vi "Simon_JKI.vi"() -> ()   [LabVIEW 2020]
uses:
  Simon Properties.ctl
  Tab Control.ctl
  <vilib>/Utility/file.llb/Read Delimited Spreadsheet (string).vi
  <vilib>/Utility/file.llb/Write Delimited Spreadsheet (string).vi
  Login Button.ctl
  Signin Button.ctl
panel:
  out "login status":string
  in  "OK":bool
  in  "Tab Control":T1
  in  "Quick Start":bool
  in  "Signin Button":T2
  in  "Login Button":T3 caption="OK Button"
  in  "Log in confirm":bool
  in  "请输入账号":string caption="Please enter your account:"
  in  "请输入密码":string caption="Please enter your password:"
  in  "请输入账号注册":string caption="Please enter your account:"
  in  "请输入密码注册":string caption="Please enter your password:"
  in  "Sign in Confirm":bool
  in  "Please enter your answer:":T4
  out "Sequence for Player to Memorize":u32(colorbox)
  out "The numbe of colors \nyou have memorized!":i32
  in  "Level Confirm":bool
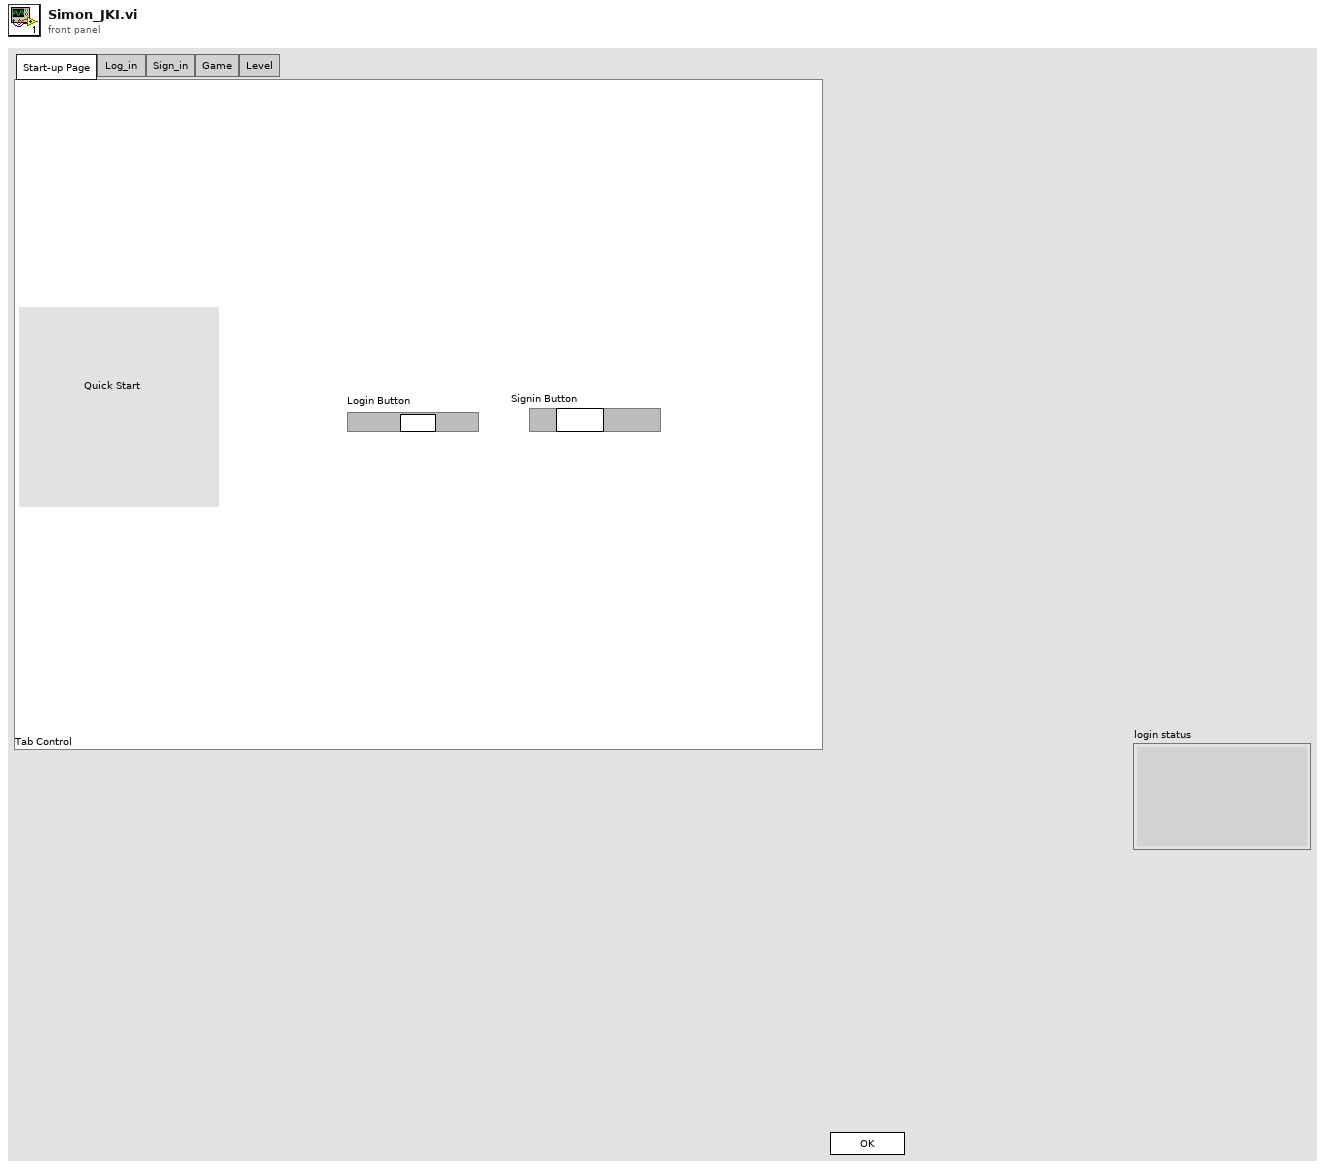
[diagram p1: front panel]
types:
  T1 = typedef "Tab Control.ctl" = enum32{"Start-up Page", "Log_in ", "Sign_in", "Game", "Level"}
  T2 = typedef "Signin Button.ctl" = bool
  T3 = typedef "Login Button.ctl" = bool
  T4 = cluster{"0":bool, "7":bool, "8":bool, "9":bool, "4":bool, "5":bool, "6":bool, "1":bool, "2":bool, "3":bool}
  T5 = enum32{"Invalid", "Standard", "Closed", "Hidden", "Minimized", "Maximized"}
  T6 = enum32{"invalid app kind", "Development System", "Run Time System", "Student Edition", "Embedded LabVIEW", "Evaluation", "Custom"}
  T7 = typedef "Simon Properties.ctl" = cluster{"Sequence ":i32[], "\n Colors":u32[], "Wait Time (ms)":u32, "Last Key":i16, "Number of Key Pressed":i32, "Record\n":i32, "Log_in":bool}
  T8 = cluster{"Core":cluster{"Current VI Reference":refnum<vi>, "Close Panel on Exit?":bool}, "Simon Properties":T7}
  T9 = cluster{"Current VI Reference":refnum<vi>, "Close Panel on Exit?":bool}
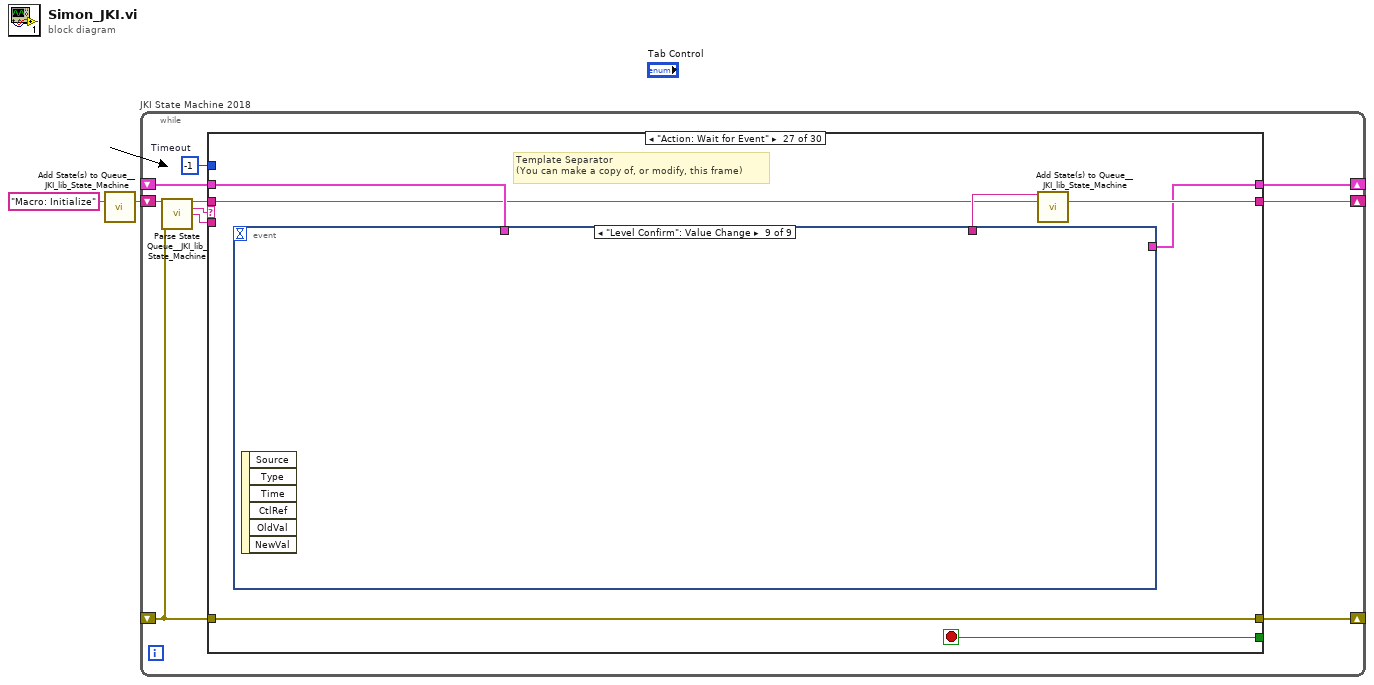
[diagram p0: block diagram]
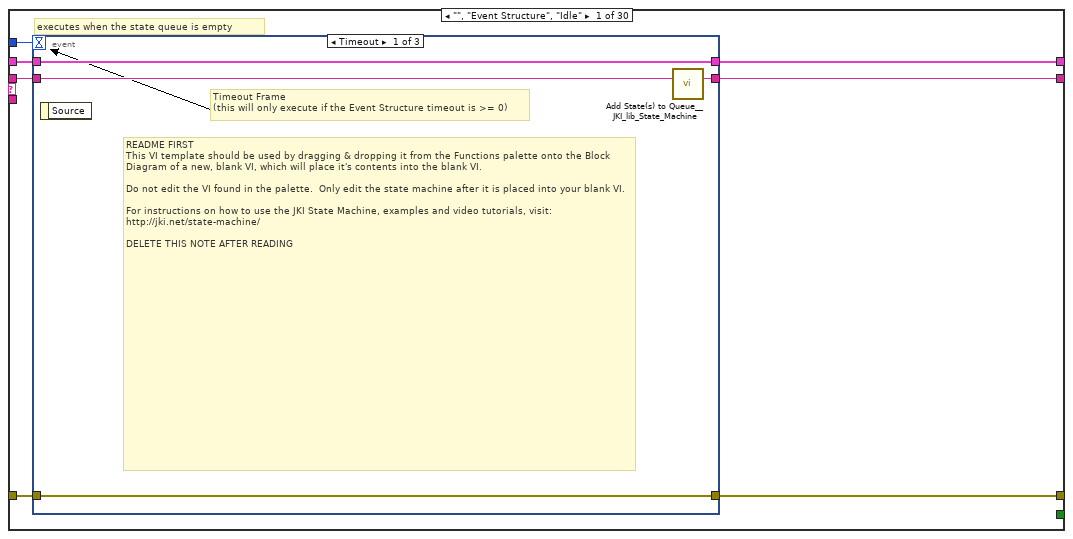
[diagram p2: hidden frame]
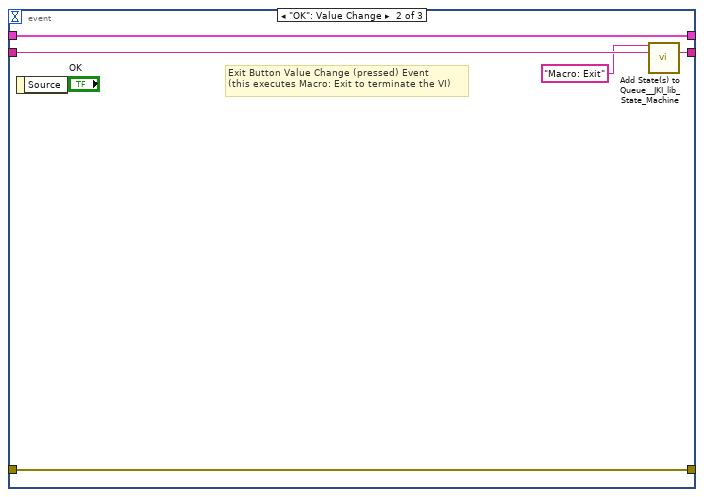
[diagram p3: hidden frame]
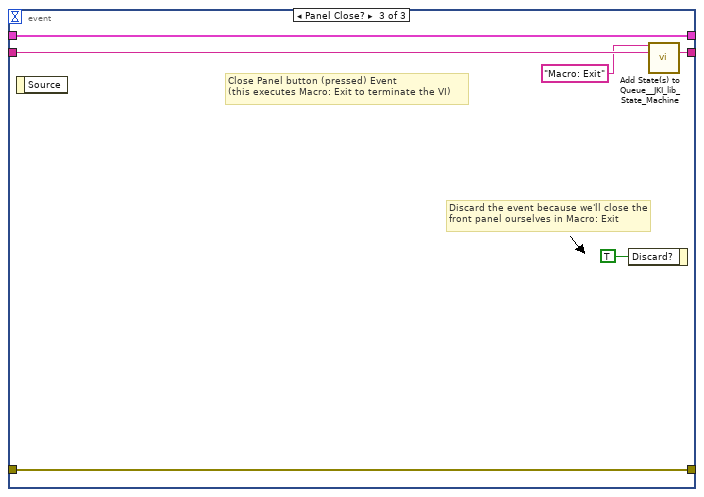
[diagram p4: hidden frame]
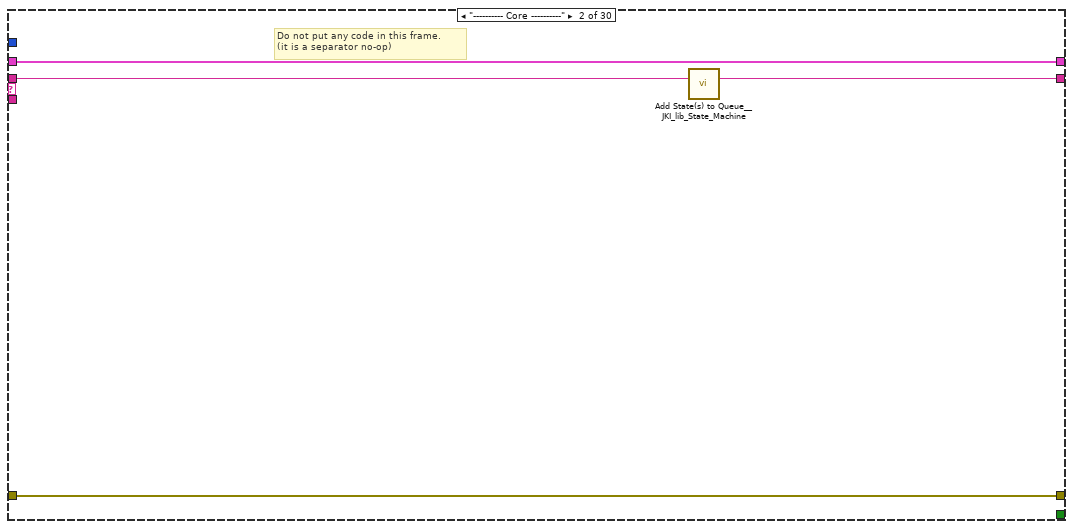
[diagram p5: hidden frame]
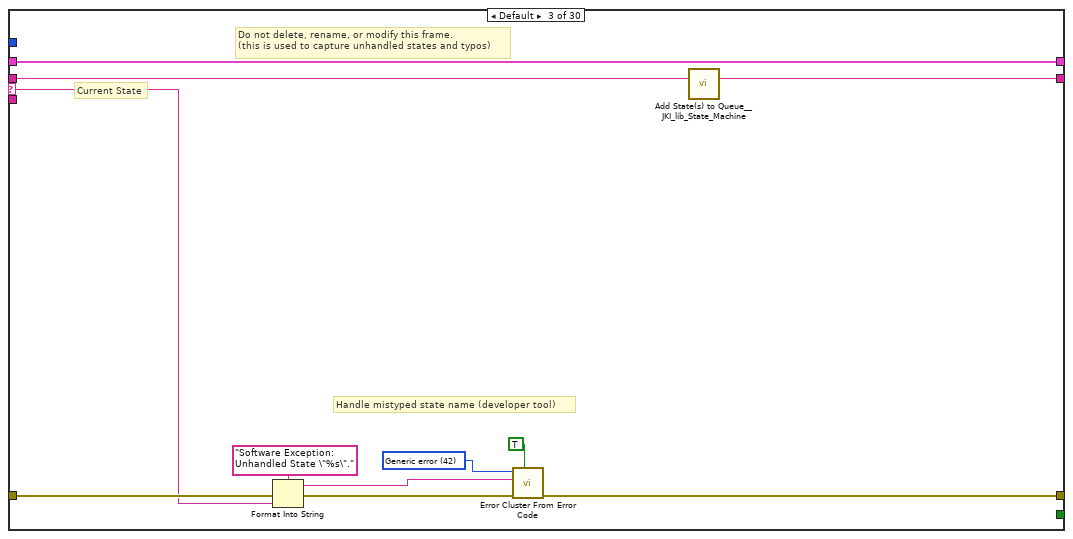
[diagram p6: hidden frame]
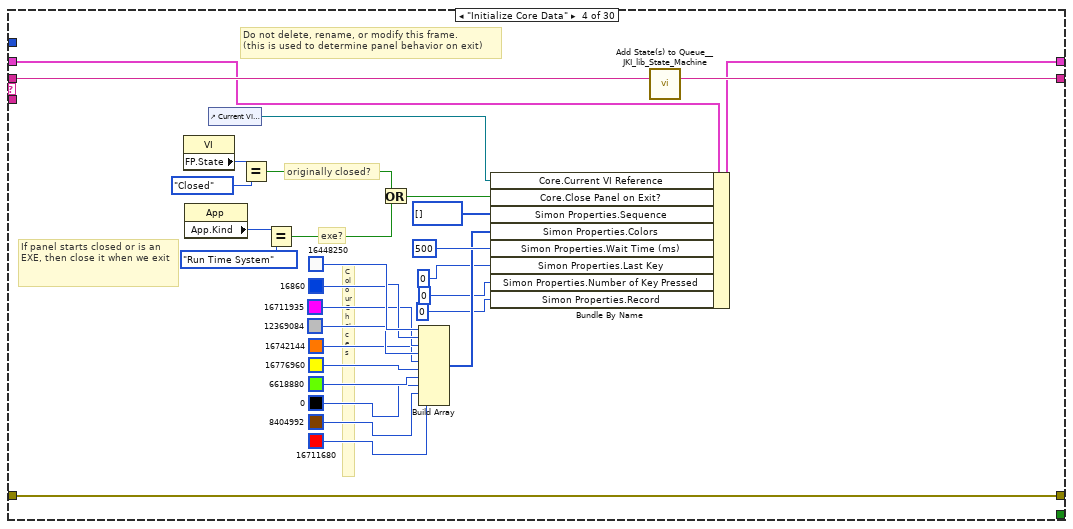
[diagram p7: hidden frame]
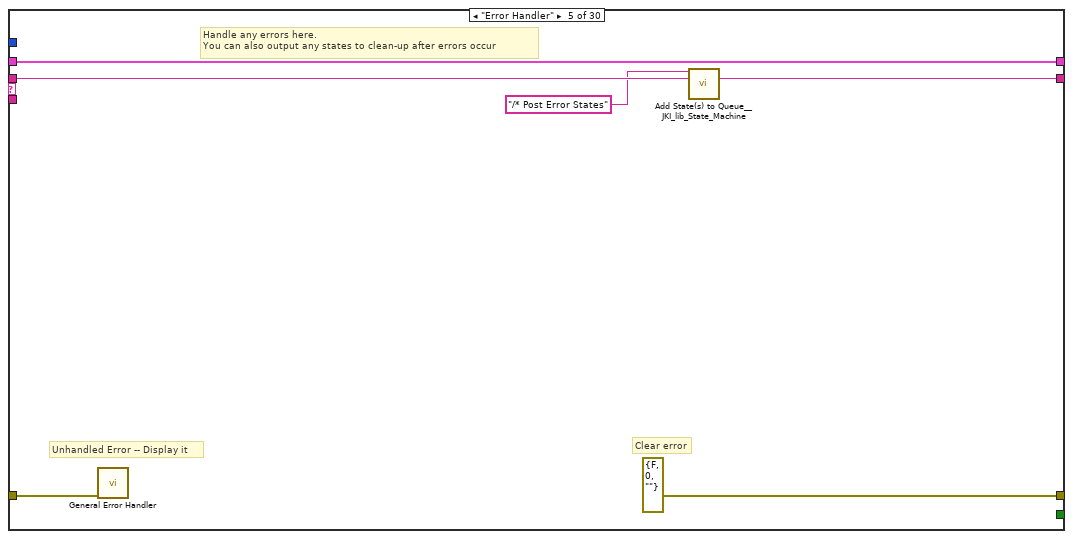
[diagram p8: hidden frame]
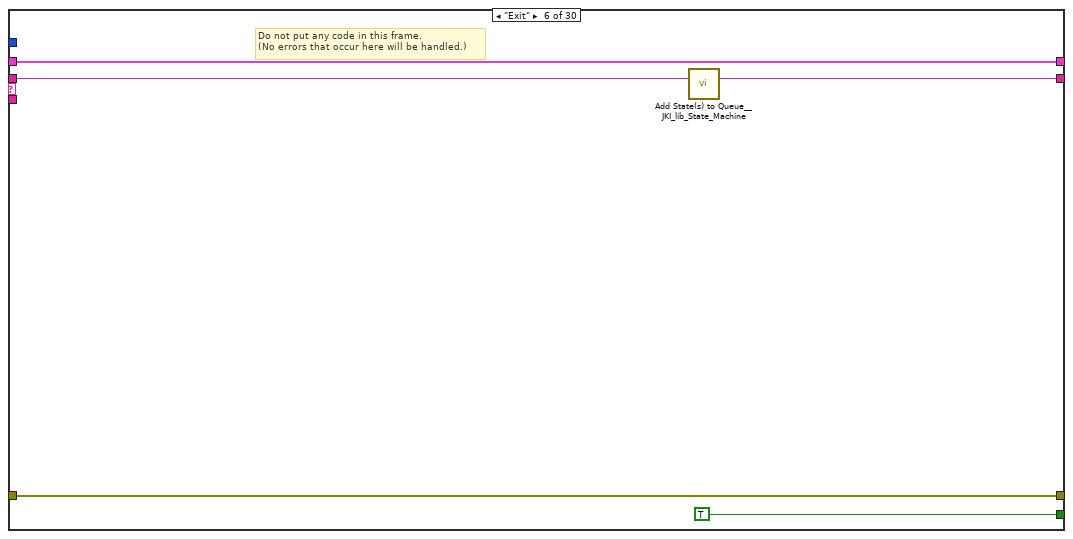
[diagram p9: hidden frame]
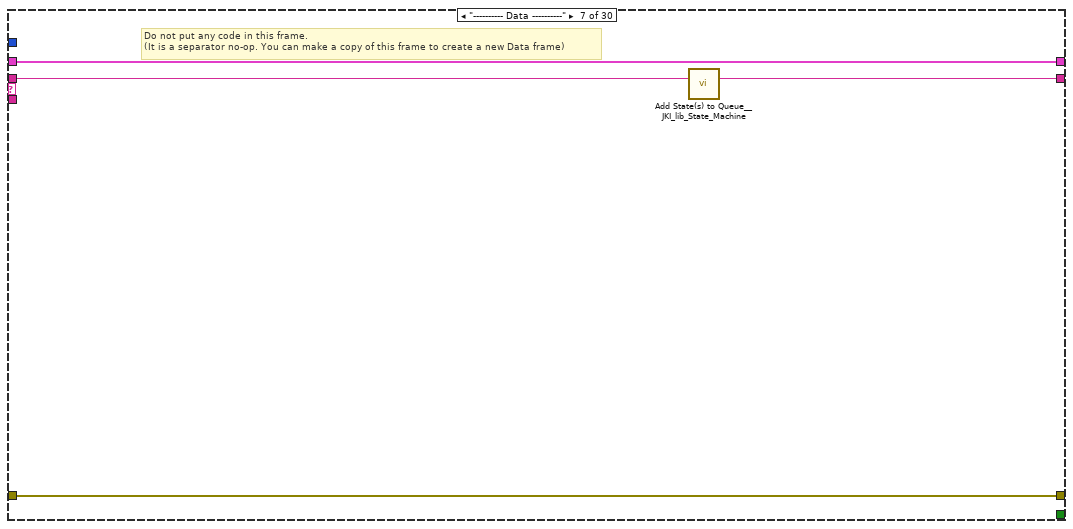
[diagram p10: hidden frame]
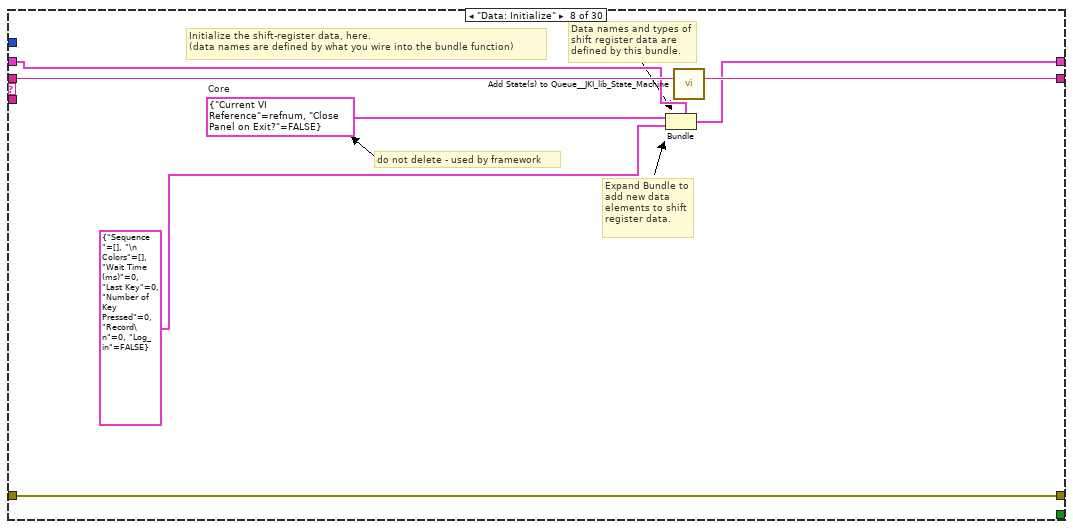
[diagram p11: hidden frame]
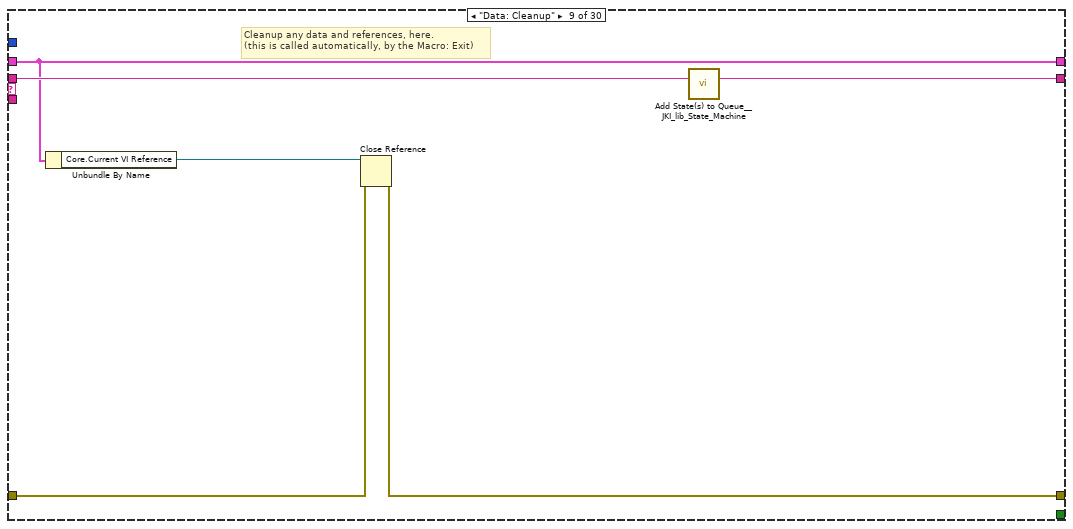
[diagram p12: hidden frame]
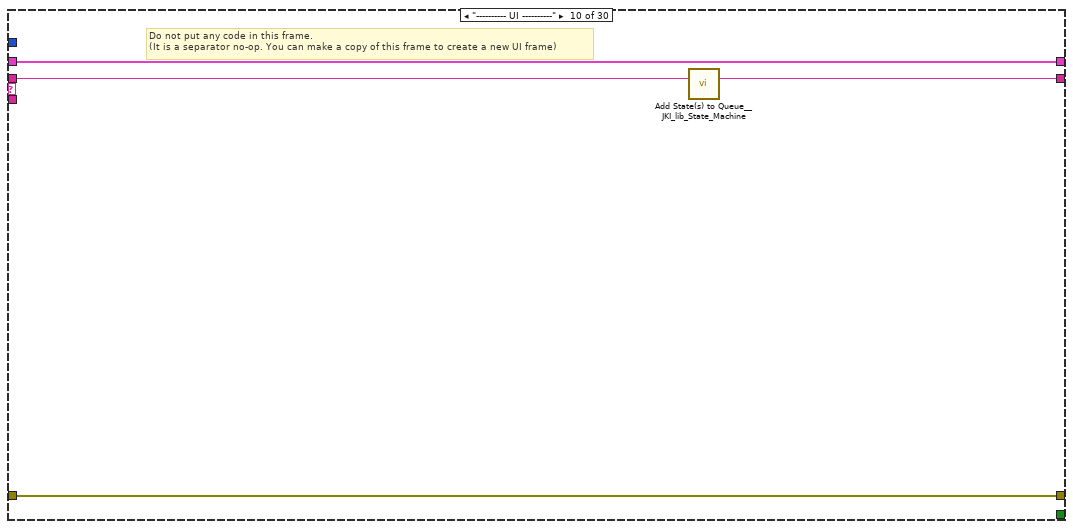
[diagram p13: hidden frame]
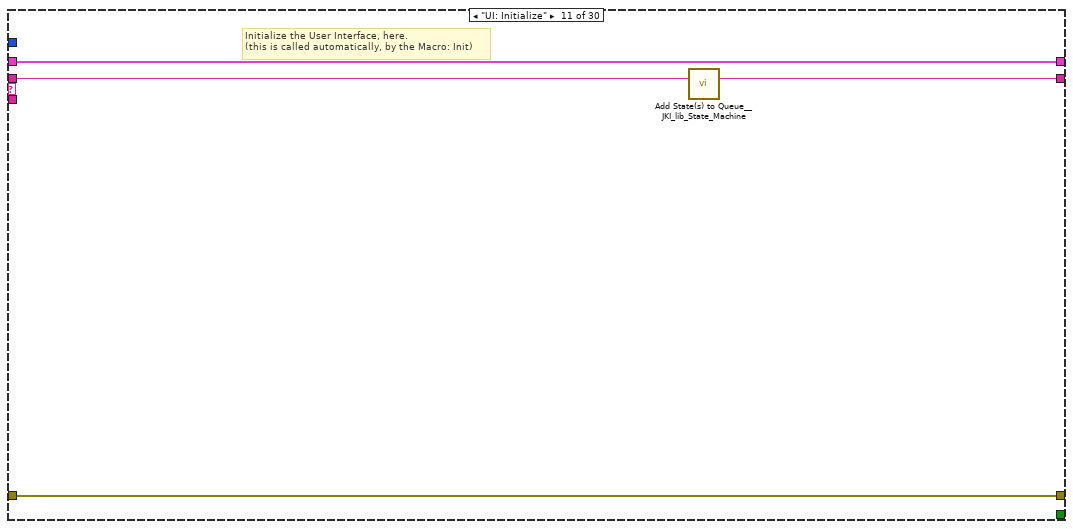
[diagram p14: hidden frame]
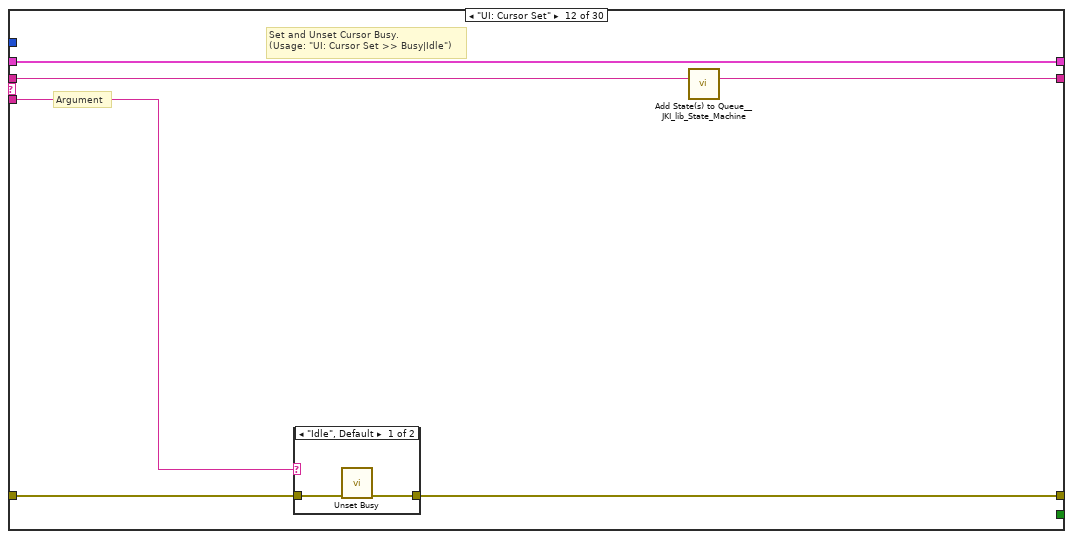
[diagram p15: hidden frame]
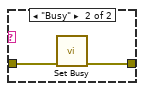
[diagram p16: hidden frame]
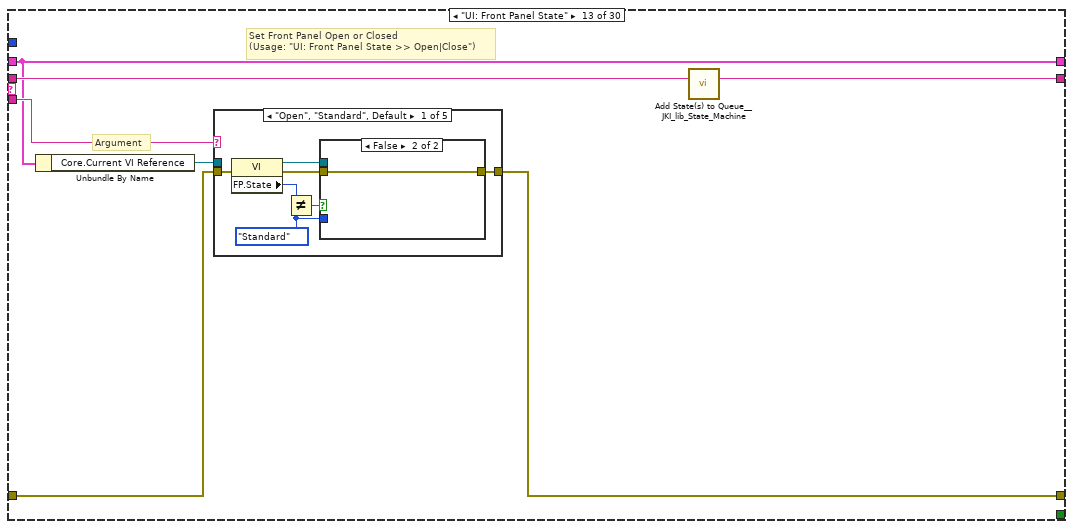
[diagram p17: hidden frame]
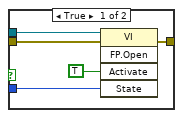
[diagram p18: hidden frame]
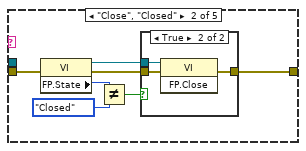
[diagram p19: hidden frame]
diagram:
  n1 = call <vilib>:"Add State(s) to Queue__JKI_lib_State_Machine.vi"("State(s) in (\"\")"="Macro: Initialize") -> ("States Out"=w2:string)  [unwired: 14 in]
  n2 = while "JKI State Machine 2018" {
    shift-right: [w6] -> _
    shift-left: _ -> [w5]
    shift-right: [w9] -> _
    shift-left: _ -> [w3]
    shift-right: [w8] -> _
    shift-left: w2 -> [w10]
    stop <- w7 stop-if-true
    w4 = -1  # Timeout
    n3 = call <vilib>:"Parse State Queue__JKI_lib_State_Machine.vi"("State Queue"=w10, "Error In (no error)"=w3) -> ("Remaining States"=w12:string, "Current State"=w13:string, "Arguments"=w11:string)  [unwired: 11 in]
    n4 = case shown="\"Action: Wait for Event\"" w13 {
      selector: w13 -> [_ _ w40 _ _ _ _ _ _ _ _ _ _ _ _ _ _ _ _ _ _ _ _ _ _ _ _ _ _ _]
      tunnel: w12 -> [w20 w39 w44 w79 w85 w90 w94 w101 w107 w111 w115 w121 w132 w196 w201 w206 w216 w220 w224 w229 w237 w243 w247 w253 w261 w284 w293 w369 w386 w394]
      tunnel: w11 -> [_ _ _ _ _ _ _ _ _ _ _ w116 w127 _ _ _ _ _ _ _ _ _ _ _ _ _ _ _ _ _]
      tunnel: w5 -> [w18 w36 w42 w58 w82 w88 w91 w96 w102 w108 w113 w119 w126 w193 w198 w203 w207 w217 w225 w231 w238 w244 w248 w254 w262 w282 w297 w371 w384 w396]
      tunnel: [w17 w37 w46 w77 errorcluster {"status"=FALSE, "code"=0, "source"=""} ("error out") w87 w92 w99 w104 w109 w112 w117 w129 w194 w199 w204 w214 w218 w222 w227 w234 w240 _ w250 w259 w281 w294 w367 w382 w393] -> w9
      tunnel: w3 -> [w16 w37 w45 w77 w81 w87 w92 w99 w105 w109 w112 w118 w130 w194 w199 w204 w214 w218 w222 w227 w234 w240 _ w250 w259 w281 w294 w367 w382 w393]
      tunnel: [w19 w38 w43 w78 w84 w89 w93 w100 w106 w110 w114 w120 w131 w195 w200 w205 w215 w219 w223 w228 w235 w241 w246 w252 w260 w283 w296 w368 w385 w395] -> w8
      tunnel: [_ _ _ _ _ TRUE _ _ _ _ _ _ _ _ _ _ _ _ _ _ _ _ _ _ _ _ _ _ _ _] -> w7
      tunnel: [w15 w36 w42 w57 w82 w88 w91 w95 w102 w108 w113 w119 w126 w193 w198 w203 w207 w217 w225 w231 w238 w244 w248 w254 w263 w282 w295 w370 w387 w396] -> w6
      tunnel: w4 -> [w14 _ _ _ _ _ _ _ _ _ _ _ _ _ _ _ _ _ _ _ _ _ _ _ _ _ _ _ _ _]
      frame "", "Event Structure", "Idle" {
        # "executes when the state queue is empty"
        n5 = event shown="[0] Timeout" {
          selector: _ -> [_ _ _]
          dyn-events: _ -> [_ _ _]
          timeout: w14 -> [_ _ _]
          tunnel: w20 -> [w24 w29 w35]
          tunnel: [w23 w28 w34] -> w19
          tunnel: w18 -> [w21 w26 w32]
          tunnel: [w22 w27 w33] -> w17
          tunnel: w16 -> [w22 w27 w33]
          tunnel: [w21 w26 w32] -> w15
          event Timeout {
            # "README FIRST\nThis VI template should be used by dragging & dropping it from the Functions palette onto the Block Diagram of a new, blank VI, which will place it's contents into the blank VI.\n\nDo not edit the VI found in the palette.  Only edit the state machine after it is placed into your blank VI.\n\nFor instructions on how to use the JKI State Machine, examples and video tutorials, visit:\nhttp://jki.net/state-machine/\n\nDELETE THIS NOTE AFTER READING"
            # "Timeout Frame\n(this will only execute if the Event Structure timeout is >= 0)"
            n6 = event-data() -> ()  [unwired: 1 in, 1 out]
            n7 = call <vilib>:"Add State(s) to Queue__JKI_lib_State_Machine.vi"("State(s) in (\"\")"=w24) -> ("States Out"=w23:string)  [unwired: 14 in]
          }
          event "OK": Value Change {
            # "Exit Button Value Change (pressed) Event\n(this executes Macro: Exit to terminate the VI)"
            n8 = event-data() -> ()  [unwired: 1 in, 1 out]
            n9 = call <vilib>:"Add State(s) to Queue__JKI_lib_State_Machine.vi"("State(s) in Front (\"\")"="Macro: Exit", "State(s) in (\"\")"=w29) -> ("States Out"=w28:string)  [unwired: 13 in]
          }
          event Panel Close? {
            # "Discard the event because we'll close the front panel ourselves in Macro: Exit"
            # "Close Panel button (pressed) Event\n(this executes Macro: Exit to terminate the VI)"
            n10 = event-data() -> ()  [unwired: 1 in, 1 out]
            n11 = event-data("Discard?"=TRUE) -> ()  [unwired: 1 in, 1 out]
            n12 = call <vilib>:"Add State(s) to Queue__JKI_lib_State_Machine.vi"("State(s) in Front (\"\")"="Macro: Exit", "State(s) in (\"\")"=w35) -> ("States Out"=w34:string)  [unwired: 13 in]
          }
        }
      }
      frame "---------- Core ----------" {
        # "Do not put any code in this frame.\n(it is a separator no-op)"
        n13 = call <vilib>:"Add State(s) to Queue__JKI_lib_State_Machine.vi"("State(s) in (\"\")"=w39) -> ("States Out"=w38:string)  [unwired: 14 in]
      }
      frame Default {
        w49 = 42 items=["No error", "Argument error", "Memory is full", "Out of zone", "End of file", "File already open", "Generic file I/O error", "File not found", "File permission error", "Disk is full", "Duplicate path", "Too many files open", "System feature not enabled", "Resource file not found", "Cannot add resource", "Resource not found", "Image not found", "Image memory error", "Pen does not exist", "Config type invalid", "Config token not found", "Config parse error", "Config memory error", "Bad external code format", "Bad external code offset", "External code not present", "Null window", "Destroy window error", "Null menu", "Print aborted", "Bad print record", "Print driver error", "Windows error during printing", "Memory error during printing", "Print dialog error", "Generic print error", "Invalid device refnum", "Device not found", "Device parameter error", "Device unit error", "Cannot open device", "Device call aborted", "Generic error", "Cancelled by user", "Object ID too low", "Object ID too high", "Object not in heap", "Unknown heap", "Unknown object (invalid DefProc)", "Unknown object (DefProc not in table)", "Message out of range", "Invalid (null) method", "Unknown message", "Manager call not supported", "Bad address", "Network operation in progress", "Network operation timed out", "Connection is busy", "Network attribute not supported", "Network error", "Address in use", "System out of memory", "Connection aborted", "Connection refused", "Not connected", "Already connected", "Connection closed", "Initialization error (interapplication manager)", "Bad occurrence", "Wait on unbound occurrence handler", "Occurrence queue overflow", "Datalog type conflict", "Unused", "Unrecognized type (interapplication manager)", "Memory corrupt", "Failed to make temporary DLL", "Old CIN version", "Drag socket not found", "Failed to load drop-object", "Failed to register OLE object", "Failed to release OLE object", "Format specifier type mismatch", "Unknown format specifier", "Too few format specifiers", "Too many format specifiers", "Scan failed", "Newer CIN version", "Error converting to variant", "Runtime menu error", "Password tampered", "Variant attribute not found", "Incompatible variant data type", "Event data is not available", "Event Store is not present", "Occurrence is not found", "Event Queue is not created", "Event info is not available", "Refnum passed is NULL", "Error retrieving Class GUID", "Error retrieving CoClass GUID", "Error retrieving TypeLib GUID.", "Bad built application magic bytes.", "Specific driver is different from the specific driver associated with the Logical Name.", "There is no session opened to the class driver.", "Max Error", "MAX - Error with config objects", "MAX - Error loading configuration", "MAX - Group not supported"]
        # "Current State"
        # "Do not delete, rename, or modify this frame.\n(this is used to capture unhandled states and typos)"
        # "Handle mistyped state name (developer tool)"
        n14 = Format Into String(format string="Software Exception: Unhandled State \"%s\"." ("message"), error in=w45, w40) -> (resulting string=w48:string, error out=w47:errorcluster)  [unwired: 1 in]
        n15 = call <vilib>:"Error Cluster From Error Code.vi"("show call chain? (False)"=TRUE, "error in (no error)"=w47, "error message (\"\")"=w48, "error code (0)"=w49) -> ("error out"=w46:errorcluster)  [unwired: 5 in]
        n16 = call <vilib>:"Add State(s) to Queue__JKI_lib_State_Machine.vi"("State(s) in (\"\")"=w44) -> ("States Out"=w43:string)  [unwired: 14 in]
      }
      frame "Initialize Core Data" {
        # "Colour Choices"
        # "Do not delete, rename, or modify this frame.\n(this is used to determine panel behavior on exit)"
        # "originally closed?"
        # "exe?"
        # "If panel starts closed or is an EXE, then close it when we exit"
        n17 = property class="VI"() -> ("FP.State"=w71:T5)  [unwired: 2 in, 2 out]
        n18 = property class="App"() -> ("App.Kind"=w76:T6)  [unwired: 2 in, 2 out]
        n19 = control-ref of="Current VI Reference"() -> (w72:refnum<vi>)
        n20 = Equal?(x=w71, y=T5."Closed" ("Front Panel Window:State")) -> (x = y?=w69:bool)
        n21 = Equal?(x=w76, y=T6."Run Time System" ("Application:Kind")) -> (x = y?=w74:bool)
        n22 = Or(x=w69, y=w74) -> (x .or. y?=w73:bool)
        n23 = Build Array(u32 16448250 ("Color Box"), u32 16860 ("Color Box"), u32 16711935 ("Color Box"), u32 12369084 ("Color Box"), u32 16742144 ("Color Box"), u32 16776960 ("Color Box"), u32 6618880 ("Color Box"), u32 0 ("Color Box"), u32 8404992 ("Color Box"), u32 16711680 ("Color Box")) -> (w54:u32[])
        n24 = Bundle By Name(cluster=w58, "Core.Current VI Reference"=w72, "Core.Close Panel on Exit?"=w73, "Simon Properties.Sequence"=i32[] [] ("Sequence"), "Simon Properties.Colors"=w54, "Simon Properties.Wait Time (ms)"=u32 500, "Simon Properties.Last Key"=i16 0, "Simon Properties.Number of Key Pressed"=0, "Simon Properties.Record"=0) -> (w57:T8)
        n25 = call <vilib>:"Add State(s) to Queue__JKI_lib_State_Machine.vi"("State(s) in (\"\")"=w79) -> ("States Out"=w78:string)  [unwired: 14 in]
      }
      frame "Error Handler" {
        # "Unhandled Error -- Display it"
        # "Handle any errors here.\nYou can also output any states to clean-up after errors occur"
        # "Clear error"
        n26 = call <vilib>:"General Error Handler.vi"("error in (no error)"=w81) -> ()  [unwired: 10 in, 5 out]
        n27 = call <vilib>:"Add State(s) to Queue__JKI_lib_State_Machine.vi"("State(s) in Front (\"\")"="/* Post Error States", "State(s) in (\"\")"=w85) -> ("States Out"=w84:string)  [unwired: 13 in]
      }
      frame "Exit" {
        # "Do not put any code in this frame.\n(No errors that occur here will be handled.)"
        n28 = call <vilib>:"Add State(s) to Queue__JKI_lib_State_Machine.vi"("State(s) in (\"\")"=w90) -> ("States Out"=w89:string)  [unwired: 14 in]
      }
      frame "---------- Data ----------" {
        # "Do not put any code in this frame.\n(It is a separator no-op. You can make a copy of this frame to create a new Data frame)"
        n29 = call <vilib>:"Add State(s) to Queue__JKI_lib_State_Machine.vi"("State(s) in (\"\")"=w94) -> ("States Out"=w93:string)  [unwired: 14 in]
      }
      frame "Data: Initialize" {
        w98 = T9 {"Current VI Reference"=refnum, "Close Panel on Exit?"=FALSE}  # Core
        # "do not delete - used by framework"
        # "Expand Bundle to add new data elements to shift register data."
        # "Data names and types of shift register data are defined by this bundle."
        # "Initialize the shift-register data, here.\n(data names are defined by what you wire into the bundle function)"
        n30 = Bundle(cluster=w96, "Core"=w98, "Simon Properties"=T7 {"Sequence "=[], "\n Colors"=[], "Wait Time (ms)"=0, "Last Key"=0, "Number of Key Pressed"=0, "Record\n"=0, "Log_in"=FALSE}) -> (w95:T8)
        n31 = call <vilib>:"Add State(s) to Queue__JKI_lib_State_Machine.vi"("State(s) in (\"\")"=w101) -> ("States Out"=w100:string)  [unwired: 14 in]
      }
      frame "Data: Cleanup" {
        # "Cleanup any data and references, here.\n(this is called automatically, by the Macro: Exit)"
        n32 = Unbundle By Name(w102) -> ("Core.Current VI Reference"=w103:refnum<vi>)
        n33 = Close Reference(reference=w103, error in (no error)=w105) -> (error out=w104:errorcluster)
        n34 = call <vilib>:"Add State(s) to Queue__JKI_lib_State_Machine.vi"("State(s) in (\"\")"=w107) -> ("States Out"=w106:string)  [unwired: 14 in]
      }
      frame "---------- UI ----------" {
        # "Do not put any code in this frame.\n(It is a separator no-op. You can make a copy of this frame to create a new UI frame)"
        n35 = call <vilib>:"Add State(s) to Queue__JKI_lib_State_Machine.vi"("State(s) in (\"\")"=w111) -> ("States Out"=w110:string)  [unwired: 14 in]
      }
      frame "UI: Initialize" {
        # "Initialize the User Interface, here.\n(this is called automatically, by the Macro: Init)"
        n36 = call <vilib>:"Add State(s) to Queue__JKI_lib_State_Machine.vi"("State(s) in (\"\")"=w115) -> ("States Out"=w114:string)  [unwired: 14 in]
      }
      frame "UI: Cursor Set" {
        # "Argument"
        # "Set and Unset Cursor Busy.\n(Usage: \"UI: Cursor Set >> Busy|Idle\")"
        n37 = case shown="\"Idle\", Default" w116 {
          tunnel: w118 -> [w123 w125]
          tunnel: [w122 w124] -> w117
          frame "Idle", Default {
            n38 = call <vilib>:"Unset Busy.vi"("error in (no error)"=w123) -> ("error out"=w122:errorcluster)  [unwired: 10 in]
          }
          frame "Busy" {
            n39 = call <vilib>:"Set Busy.vi"("error in (no error)"=w125) -> ("error out"=w124:errorcluster)  [unwired: 9 in, 1 out]
          }
        }
        n40 = call <vilib>:"Add State(s) to Queue__JKI_lib_State_Machine.vi"("State(s) in (\"\")"=w121) -> ("States Out"=w120:string)  [unwired: 14 in]
      }
      frame "UI: Front Panel State" {
        # "Argument"
        # "Set Front Panel Open or Closed\n(Usage: \"UI: Front Panel State >> Open|Close\")"
        n41 = Unbundle By Name(w126) -> ("Core.Current VI Reference"=w128:refnum<vi>)
        n42 = case shown="\"Open\", \"Standard\", Default" w127 {
          tunnel: w130 -> [w138 w151 w162 w174 w186]
          tunnel: [w139 w152 w163 w175 w187] -> w129
          tunnel: w128 -> [_ _ _ _ _]
          frame "Open", "Standard", Default {
            w133 = T5."Standard" ("State")
            n43 = property class="VI"(error in=w138) -> (reference out=w136:refnum<vi>, error out=w137:errorcluster, "FP.State"=w135:T5)  [unwired: 1 in]
            n44 = Not Equal?(x=w135, y=w133) -> (x != y?=w134:bool)
            n45 = case shown="False" w134 {
              tunnel: [w143 w145] -> w139
              tunnel: w137 -> [w142 w145]
              tunnel: w136 -> [w141 _]
              tunnel: w133 -> [w140 _]
              frame True {
                n46 = invoke class="VI" method="FP.Open"(reference=w141, error in=w142, "Activate"=TRUE, "State"=w140) -> (error out=w143:errorcluster)  [unwired: 1 in, 4 out]
              }
              frame False {
              }
            }
          }
          frame "Close", "Closed" {
            n47 = property class="VI"(error in=w151) -> (reference out=w149:refnum<vi>, error out=w150:errorcluster, "FP.State"=w147:T5)  [unwired: 1 in]
            n48 = Not Equal?(x=w147, y=T5."Closed" ("Front Panel Window:State")) -> (x != y?=w146:bool)
            n49 = case shown="True" w146 {
              tunnel: [w153 w156] -> w152
              tunnel: w150 -> [w153 w155]
              tunnel: w149 -> [_ w154]
              frame False {
              }
              frame True {
                n50 = invoke class="VI" method="FP.Close"(reference=w154, error in=w155) -> (error out=w156:errorcluster)  [unwired: 1 in, 2 out]
              }
            }
          }
          frame "Hidden", "Hide" {
            w157 = T5."Hidden" ("State")
            n51 = property class="VI"(error in=w162) -> (reference out=w160:refnum<vi>, error out=w161:errorcluster, "FP.State"=w159:T5)  [unwired: 1 in]
            n52 = Not Equal?(x=w159, y=w157) -> (x != y?=w158:bool)
            n53 = case shown="True" w158 {
              tunnel: [w167 w168] -> w163
              tunnel: w161 -> [w166 w168]
              tunnel: w160 -> [w165 _]
              tunnel: w157 -> [w164 _]
              frame True {
                n54 = invoke class="VI" method="FP.Open"(reference=w165, error in=w166, "State"=w164) -> (error out=w167:errorcluster)  [unwired: 2 in, 4 out]
              }
              frame False {
              }
            }
          }
          frame "Minimize", "Minimized" {
            w169 = T5."Minimized" ("State")
            n55 = property class="VI"(error in=w174) -> (reference out=w172:refnum<vi>, error out=w173:errorcluster, "FP.State"=w171:T5)  [unwired: 1 in]
            n56 = Not Equal?(x=w171, y=w169) -> (x != y?=w170:bool)
            n57 = case shown="True" w170 {
              tunnel: [w179 w180] -> w175
              tunnel: w173 -> [w178 w180]
              tunnel: w172 -> [w177 _]
              tunnel: w169 -> [w176 _]
              frame True {
                n58 = invoke class="VI" method="FP.Open"(reference=w177, error in=w178, "State"=w176) -> (error out=w179:errorcluster)  [unwired: 2 in, 4 out]
              }
              frame False {
              }
            }
          }
          frame "Maximize", "Maximized" {
            w181 = T5."Maximized" ("State")
            n59 = property class="VI"(error in=w186) -> (reference out=w184:refnum<vi>, error out=w185:errorcluster, "FP.State"=w183:T5)  [unwired: 1 in]
            n60 = Not Equal?(x=w183, y=w181) -> (x != y?=w182:bool)
            n61 = case shown="True" w182 {
              tunnel: [w191 w192] -> w187
              tunnel: w185 -> [w190 w192]
              tunnel: w184 -> [w189 _]
              tunnel: w181 -> [w188 _]
              frame True {
                n62 = invoke class="VI" method="FP.Open"(reference=w189, error in=w190, "State"=w188) -> (error out=w191:errorcluster)  [unwired: 2 in, 4 out]
              }
              frame False {
              }
            }
          }
        }
        n63 = call <vilib>:"Add State(s) to Queue__JKI_lib_State_Machine.vi"("State(s) in (\"\")"=w132) -> ("States Out"=w131:string)  [unwired: 14 in]
      }
      frame "---------- Macro ----------" {
        # "Do not put any code in this frame.\n(It is a separator no-op. You can make a copy of this frame to create a new Macro frame)"
        n64 = call <vilib>:"Add State(s) to Queue__JKI_lib_State_Machine.vi"("State(s) in (\"\")"=w196) -> ("States Out"=w195:string)  [unwired: 14 in]
      }
      frame "Macro: Initialize" {
        # "Initialization Macro\n(This is called once, when the VI starts)"
        n65 = call <vilib>:"Add State(s) to Queue__JKI_lib_State_Machine.vi"("State(s) in Front (\"\")"="Data: Initialize\nInitialize Core Data\nUI: Initialize\nUI: Front Panel State >> Open\nAction: Switch to Start-up Page", "State(s) in (\"\")"=w201) -> ("States Out"=w200:string)  [unwired: 13 in]
      }
      frame "Macro: Qucik Start Flow" {
        w202 = "Data: Initialize\nInitialize Core Data\nUI: Initialize\nUI: Front Panel State >> Open"  # Data: Initialize Initialize Core Data UI: Initialize UI: Front Panel State >> Open
        # "Do not put any code in this frame.\n(It is a separator no-op. You can make a copy of this frame to create a new Macro frame)"
        n66 = call <vilib>:"Add State(s) to Queue__JKI_lib_State_Machine.vi"("State(s) in Front (\"\")"=w202, "State(s) in (\"\")"=w206) -> ("States Out"=w205:string)  [unwired: 13 in]
      }
      frame "Macro: Exit" {
        # "Exit Macro\n(This is called once, when the VI exits)"
        n67 = Unbundle By Name(w207) -> ("Core.Close Panel on Exit?"=w208:bool)
        n68 = Select(t="UI: Front Panel State >> Close", s=w208, f="") -> (s? t:f=w211:string)
        n69 = call <vilib>:"Add State(s) to Queue__JKI_lib_State_Machine.vi"("State(s) in (\"\")"=w211, "State(s) at Back (\"\")"="Data: Cleanup\nExit") -> ("States Out"=w209:string)  [unwired: 13 in]
        n70 = call <vilib>:"Add State(s) to Queue__JKI_lib_State_Machine.vi"("State(s) in Front (\"\")"=w209, "State(s) in (\"\")"=w216) -> ("States Out"=w215:string)  [unwired: 13 in]
      }
      frame "---------- Action ----------" {
        # "Your code here.\n(You can make a copy of, or modify, this frame)"
        n71 = call <vilib>:"Add State(s) to Queue__JKI_lib_State_Machine.vi"("State(s) in (\"\")"=w220) -> ("States Out"=w219:string)  [unwired: 14 in]
      }
      frame "Action: Switch to Start-up Page" {
        # "Press Quick Start Button to start the game directly"
        n72 = local write "Tab Control"(Tab_Control."Start-up Page" ("Tab Control")) -> ()
        n73 = call <vilib>:"Add State(s) to Queue__JKI_lib_State_Machine.vi"("State(s) in Front (\"\")"="Action: Wait for Event" ("State(s) in Front (\"\")"), "State(s) in (\"\")"=w224) -> ("States Out"=w223:string)  [unwired: 13 in]
      }
      frame "Action: Switch to Login Page" {
        n74 = local write "Tab Control"(Tab_Control."Log_in " ("Tab Control")) -> ()
        n75 = call <vilib>:"Add State(s) to Queue__JKI_lib_State_Machine.vi"("State(s) in Front (\"\")"="Action: Wait for Event" ("State(s) in Front (\"\")"), "State(s) in (\"\")"=w229) -> ("States Out"=w228:string)  [unwired: 13 in]
      }
      frame "Action: Switch to Signin Page" {
        n76 = local write "Tab Control"(Tab_Control."Sign_in" ("Tab Control")) -> ()
        n77 = call <vilib>:"Add State(s) to Queue__JKI_lib_State_Machine.vi"("State(s) in Front (\"\")"="Action: Wait for Event" ("State(s) in Front (\"\")"), "State(s) in (\"\")"=w237) -> ("States Out"=w235:string)  [unwired: 13 in]
      }
      frame "Action: Switch to Game Page" {
        n78 = local write "Tab Control"(Tab_Control."Game" ("Tab Control")) -> ()
        n79 = call <vilib>:"Add State(s) to Queue__JKI_lib_State_Machine.vi"("State(s) in Front (\"\")"="Action: Add New Color" ("State(s) in Front (\"\")"), "State(s) in (\"\")"=w243) -> ("States Out"=w241:string)  [unwired: 13 in]
      }
      frame "Action: Switch to Level Page" {
        n80 = local write "Tab Control"(Tab_Control."Level" ("Tab Control")) -> ()
        n81 = call <vilib>:"Add State(s) to Queue__JKI_lib_State_Machine.vi"("State(s) in Front (\"\")"="Action: Level Select " ("State(s) in Front (\"\")"), "State(s) in (\"\")"=w247) -> ("States Out"=w246:string)  [unwired: 13 in]
      }
      frame "Action: Register Successfully" {
        n82 = flat-sequence {
          tunnel: ["Action: Switch to Login Page" ("State(s) in Front (\"\")")] -> w251
          frame #0 {
            n83 = Wait (ms)(milliseconds to wait=u32 1000) -> ()  [unwired: 1 out]
            n84 = One Button Dialog(message="You have registered successfully!") -> ()  [unwired: 1 in, 1 out]
          }
          frame #1 {
          }
        }
        n85 = call <vilib>:"Add State(s) to Queue__JKI_lib_State_Machine.vi"("State(s) in Front (\"\")"=w251, "State(s) in (\"\")"=w253) -> ("States Out"=w252:string)  [unwired: 13 in]
      }
      frame "Action: Add New Color" {
        # "Your code here.\n(You can make a copy of, or modify, this frame)"
        n86 = Unbundle By Name(w262) -> ("Simon Properties.Sequence"=w258:i32[], "Simon Properties.Colors"=w264:u32[])
        n87 = local write "Tab Control"(Tab_Control."Game" ("Tab Control")) -> ()
        n88 = while {
          tunnel: w258 -> [w271]
          tunnel: w264 -> [w270]
          tunnel: [w272] -> w265
          stop <- w273 stop-if-true
          # "Generate new color"
          # "Acquire the last state"
          n89 = Random Number (0-1)() -> (number: 0 to 1=w278:dbl)
          n90 = Reverse 1D Array(array=w271) -> (reversed array=w280:i32[])
          n91 = Array Size(array=w270) -> (size(s)=w276:i32)
          n92 = Index Array(array=w280, index=0) -> (element=w269:i32)
          n93 = To Double Precision Float(number=w276) -> (double precision float=w275:dbl)
          n94 = Multiply(x=w275, y=w278) -> (x*y=w277:dbl)
          n95 = Round Toward -Infinity(1:w277) -> (0:w274:dbl)
          n96 = To Long Integer(number=w274) -> (32bit integer=w272:i32)
          n97 = Not Equal?(x=w269, y=w272) -> (x != y?=w273:bool)
        }
        n98 = Build Array (concatenate)(w258, w265) -> (w266:i32[])
        n99 = Bundle By Name(cluster=w262, "Simon Properties.Sequence"=w266) -> (w263:T8)
        n100 = call <vilib>:"Add State(s) to Queue__JKI_lib_State_Machine.vi"("State(s) in Front (\"\")"="Action: Show Sequence" ("State(s) in Front (\"\")"), "State(s) in (\"\")"=w261) -> ("States Out"=w260:string)  [unwired: 13 in]
      }
      frame "Action: Show Sequence" {
        # "Your code here.\n(You can make a copy of, or modify, this frame)"
        n101 = Unbundle By Name(w282) -> ("Simon Properties.Colors"=w285:u32[], "Simon Properties.Sequence"=w286:i32[], "Simon Properties.Wait Time (ms)"=w287:u32)
        n102 = for {
          tunnel: w285 -> [w292]
          tunnel: w286 -> [w291] mode=indexing
          tunnel: w287 -> [w289]
          n103 = Index Array(array=w292, index=w291) -> (element=→"Sequence for Player to Memorize":u32)
          n104 = Wait (ms)(milliseconds to wait=w289) -> ()  [unwired: 1 out]
        }
        n105 = call <vilib>:"Add State(s) to Queue__JKI_lib_State_Machine.vi"("State(s) in Front (\"\")"="Action: Wait for Event" ("State(s) in Front (\"\")"), "State(s) in (\"\")"=w284) -> ("States Out"=w283:string)  [unwired: 13 in]
      }
      frame "Action: Wait for Event" {
        # "Template Separator\n(You can make a copy of, or modify, this frame)"
        n106 = event shown="[8] \"Level Confirm\": Value Change" {
          selector: _ -> [_ _ _ _ _ _ _ _ _]
          dyn-events: _ -> [_ _ _ _ _ _ _ _ _]
          timeout: _ -> [_ _ _ _ _ _ _ _ _]
          tunnel: [w299 w302 w316 w323 w327 w328 w347 w364 _] -> w295
          tunnel: ["Macro: Exit" ("State(s) in Front (\"\")") w304 "Action: Check" ("State(s) in Front (\"\")") "Action: Add New Color" ("State(s) in Front (\"\")") "Action: Switch to Login Page" ("State(s) in Front (\"\")") w329 "Action: Register Successfully" ("State(s) in Front (\"\")") "Action: Switch to Signin Page" ("State(s) in Front (\"\")") _] -> w298
          tunnel: w297 -> [w299 w303 w314 w323 w327 w328 w347 w364 _]
          event Panel Close? {
            n107 = event-data() -> ()  [unwired: 1 in, 1 out]
            n108 = event-data("Discard?"=TRUE) -> ()  [unwired: 1 in, 1 out]
          }
          event Key Down {
            # "Keyboard input, one value at a time"
            # "48-57"
            n109 = event-data() -> ("Char"=w305:i16)  [unwired: 1 in]
            n110 = case shown="Default" w305 {
              selector: w305 -> [_ w312]
              tunnel: [w306 w313] -> w302
              tunnel: ["Action: Wait for Event" ("State(s) in Front (\"\")") "Action: Check" ("State(s) in Front (\"\")")] -> w304
              tunnel: w303 -> [w306 w308]
              frame Default {
              }
              frame 48..57 {
                # "The purpose of recording the last key is to see if it aligns with the sequence."
                # "0-9 represents 10 colors"
                n111 = Subtract(x=w312, y=i16 48) -> (x-y=w310:i16)
                n112 = Bundle By Name(cluster=w308, "Simon Properties.Last Key"=w310) -> (w313:T8)
              }
            }
          }
          event "Please enter your answer:": Value Change {
            # "Mouse click input, one value at a time"
            n113 = event-data() -> ()  [unwired: 1 in, 6 out]
            n114 = Cluster To Array(cluster="Please enter your answer:") -> (array=w321:bool[])
            n115 = Boolean Array To Number(Boolean array=w321) -> (number=w320:u32)
            n116 = To Double Precision Float(number=w320) -> (double precision float=w319:dbl)
            n117 = Logarithm Base 2(1:w319) -> (0:w318:dbl)
            n118 = To Word Integer(number=w318) -> (16bit integer=w317:i16)
            n119 = Bundle By Name(cluster=w314, "Simon Properties.Last Key"=w317) -> (w316:T8)
          }
          event "Quick Start": Value Change {
            n120 = event-data() -> ()  [unwired: 1 in, 6 out]
            n121 = local write "Tab Control"(Tab_Control."Game" ("Tab Control")) -> ()
          }
          event Value Change {
            n122 = event-data() -> ()  [unwired: 1 in, 6 out]
          }
          event "Log in confirm": Value Change {
            n123 = event-data() -> ()  [unwired: 1 in, 6 out]
            n124 = call <vilib>:"Application Directory.vi"() -> ("Application Directory"=w331:path)
            n125 = Build Path(base path=w331, name or relative path=path "Userinfo.csv") -> (appended path=w334:path)
            n126 = call-poly <vilib>:"Read Delimited Spreadsheet.vi"("file path (dialog if empty)"=w334, "transpose? (F)"=TRUE, "delimiter (\\t)"="," ("delimiter (\\t)")) -> ("all rows"=w330:string[][])  [unwired: 7 in, 5 out]
            n127 = while {
              tunnel: w330 -> [w340] mode=indexing
              tunnel: [w339] -> w329
              stop <- w336 stop-if-true
              n128 = Index Array(array=w340) -> (element #1=w338:string, element #2=w337:string)  [unwired: 2 in]
              n129 = Equal?(x="请输入账号", y=w338) -> (x = y?=w346:bool)
              n130 = Equal?(x=w337, y="请输入密码") -> (x = y?=w345:bool)
              n131 = And(x=w346, y=w345) -> (x .and. y?=w336:bool)
              n132 = Select(t="Action: Switch to Start-up Page", s=w336, f="Action: Switch to Start-up Page ") -> (s? t:f=w339:string)
              "login status" <- w339
            }
          }
          event "Sign in Confirm": Value Change {
            n133 = event-data() -> ()  [unwired: 1 in, 6 out]
            n134 = call <vilib>:"Application Directory.vi"() -> ("Application Directory"=w352:path)
            n135 = Build Path(base path=w352, name or relative path=path "Userinfo.csv") -> (appended path=w351:path)
            n136 = call-poly <vilib>:"Read Delimited Spreadsheet.vi"("file path (dialog if empty)"=w351, "transpose? (F)"=TRUE, "delimiter (\\t)"="," ("delimiter (\\t)")) -> ("all rows"=w353:string[][])  [unwired: 7 in, 5 out]
            n137 = Transpose 2D Array(2D array=w353) -> (transposed array=w363:string[][])
            n138 = Index Array(array=w363) -> (element #1=w362:string[], element #2=w361:string[])  [unwired: 4 in]
            n139 = Insert Into Array(array=w361, new element="请输入密码注册") -> (w359:string[])  [unwired: 1 in]
            n140 = Insert Into Array(array=w362, new element="请输入账号注册") -> (w360:string[])  [unwired: 1 in]
            n141 = Build Array(w360, w359) -> (w358:string[][])
            n142 = call-poly <vilib>:"Write Delimited Spreadsheet.vi"("file path (dialog if empty)"=w351, "2D data"=w358, "delimiter (\\t)"="," ("delimiter (\\t)")) -> ()  [unwired: 11 in, 2 out]
          }
          event Value Change {
            n143 = event-data() -> ()  [unwired: 1 in, 6 out]
            n144 = local write "Tab Control"(Tab_Control."Sign_in" ("Tab Control")) -> ()
          }
          event "Level Confirm": Value Change {
            n145 = event-data() -> ()  [unwired: 1 in, 6 out]
          }
        }
        n146 = call <vilib>:"Add State(s) to Queue__JKI_lib_State_Machine.vi"("State(s) in Front (\"\")"=w298, "State(s) in (\"\")"=w293) -> ("States Out"=w296:string)  [unwired: 13 in]
      }
      frame "Action: Check" {
        # "Template Separator\n(You can make a copy of, or modify, this frame)"
        n147 = Unbundle By Name(w371) -> ("Simon Properties.Sequence"=w374:i32[], "Simon Properties.Number of Key Pressed"=w372:i32, "Simon Properties.Last Key"=w375:i16)
        n148 = Array Size(array=w374) -> (size(s)=w373:i32)
        n149 = To Long Integer(number=w375) -> (32bit integer=w376:i32)
        n150 = Increment(x=w372) -> (x+1=w381:i32)
        n151 = Index Array(array=w374, index=w372) -> (element=w377:i32)
        n152 = Equal?(x=w373, y=w381) -> (x = y?=w378:bool)
        n153 = Equal?(x=w377, y=w376) -> (x = y?=w379:bool)
        n154 = call "Enter finished"("Display result?"=w379, "Enter finished?"=w378) -> ("Enter finshed?"=w380:string)  [unwired: 9 in]
        n155 = Bundle By Name(cluster=w371, "Simon Properties.Number of Key Pressed"=w381) -> (w370:T8)
        n156 = call <vilib>:"Add State(s) to Queue__JKI_lib_State_Machine.vi"("State(s) in Front (\"\")"=w380, "State(s) in (\"\")"=w369) -> ("States Out"=w368:string)  [unwired: 13 in]
      }
      frame "Action: Success" {
        # "Reset the number of key pressed to see if every time the input is correct."
        # "Template Separator\n(You can make a copy of, or modify, this frame)"
        n157 = Unbundle By Name(w384) -> ("Simon Properties.Record"=w383:i32)
        n158 = Increment(x=w383) -> (x+1=w390:i32)
        "The numbe of colors \nyou have memorized!" <- w390
        n159 = One Button Dialog(message="Excellent! Let's add one more to the sequence") -> ()  [unwired: 1 in, 1 out]
        n160 = Bundle By Name(cluster=w384, "Simon Properties.Record"=w390, "Simon Properties.Number of Key Pressed"=0, "Simon Properties.Wait Time (ms)"=u32 500 ("Wait Time (ms)")) -> (w387:T8)
        n161 = call <vilib>:"Add State(s) to Queue__JKI_lib_State_Machine.vi"("State(s) in Front (\"\")"="Action: Add New Color" ("State(s) in Front (\"\")"), "State(s) in (\"\")"=w386) -> ("States Out"=w385:string)  [unwired: 13 in]
      }
      frame "Action: Fail" {
        # "Template Separator\n(You can make a copy of, or modify, this frame)"
        n162 = Unbundle By Name(w396) -> ("Simon Properties.Number of Key Pressed"=w400:i32, "Simon Properties.Sequence"=w402:i32[])
        n163 = Decrement(x=w400) -> (x-1=w401:i32)
        n164 = Index Array(array=w402, index=w401) -> (element=w403:i32)
        n165 = case shown="8" w403 {
          tunnel: ["White" "Blue" "Pink" "Gray" "Orange" "Yellow" "GREEN" "Black" "Brown" "Red"] -> w397
          frame 0, Default {
          }
          frame 1 {
          }
          frame 2 {
          }
          frame 3 {
          }
          frame 4 {
          }
          frame 5 {
          }
          frame 6 {
          }
          frame 7 {
          }
          frame 8 {
          }
          frame 9 {
          }
        }
        n166 = Format Into String(format string="Bad luck! You memorised a sequence %d long. \nThe correct colour was %s." ("message"), w401, w397) -> (resulting string=w398:string)  [unwired: 2 in, 1 out]
        n167 = call <vilib>:"Add State(s) to Queue__JKI_lib_State_Machine.vi"("State(s) in Front (\"\")"="Macro: Initialize" ("State(s) in Front (\"\")"), "State(s) in (\"\")"=w394) -> ("States Out"=w395:string)  [unwired: 13 in]
        n168 = One Button Dialog(message=w398) -> ()  [unwired: 1 in, 1 out]
      }
    }
  }
